vi "BuildConfigurationFilePaths.vi"(0 "name or relative path":string="Report Cummulative") -> (4 "Base Path":path=path "C:/Minda", 6 "User Configuration":path=path "C:/Minda/Configuration Files/UserConfiguration.usr", 8 "Product Configuration":path=path "C:/Minda/Configuration Files/ProductConfiguration.pdt", 10 "HWIO Configuration":path=path "C:/Minda/Configuration Files/HWIOConfiguration.txt", 14 "System File Path":path=path "C:/Minda/A-0090-System.bin" caption="System Verify")   [LabVIEW 2015]
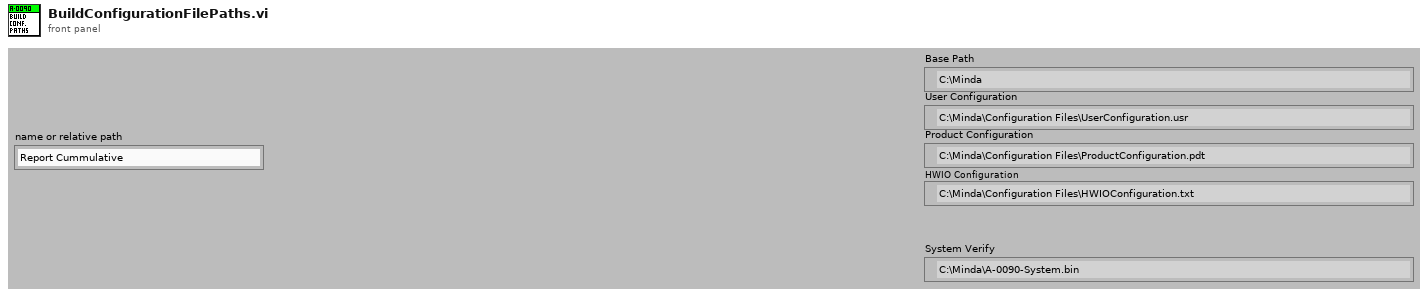
[diagram p1: front panel]
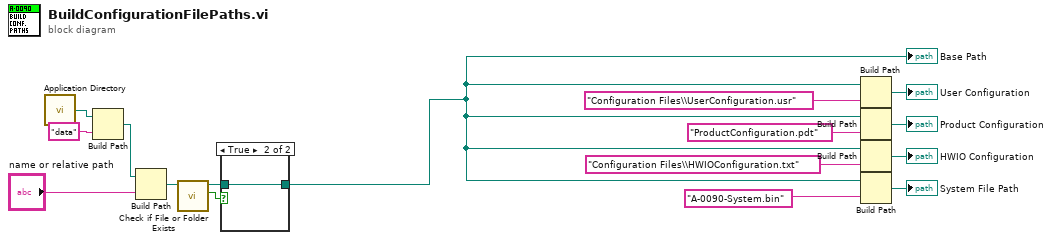
[diagram p0: block diagram]
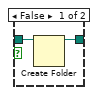
[diagram p2: hidden frame]
diagram:
  n1 = call <vilib>:"Application Directory.vi"() -> ("Application Directory"=w3:path)
  n2 = Build Path(base path=w3, name or relative path="data") -> (appended path=w2:path)
  n3 = Build Path(base path=w2, name or relative path="name or relative path") -> (appended path=w6:path)
  n4 = call <vilib>:"Check if File or Folder Exists.vi"("path"=w6) -> ("file or folder exists?"=w5:bool, "dup path"=w4:path)  [unwired: 8 in, 1 out]
  n5 = case shown="True" w5 {
    tunnel: w4 -> [w18 w19]
    tunnel: [w17 w19] -> w1
    frame False {
      n6 = Create Folder(path (use dialog)=w18) -> (created path=w17:path)  [unwired: 2 in, 2 out]
    }
    frame True {
    }
  }
  "Base Path" <- w1
  n7 = Build Path(base path=w1, name or relative path="Configuration Files\\UserConfiguration.usr" ("string")) -> (appended path=→"User Configuration":path)
  n8 = Build Path(base path=w1, name or relative path="ProductConfiguration.pdt" ("string")) -> (appended path=→"Product Configuration":path)
  n9 = Build Path(base path=w1, name or relative path="Configuration Files\\HWIOConfiguration.txt" ("string")) -> (appended path=→"HWIO Configuration":path)
  n10 = Build Path(base path=w1, name or relative path="A-0090-System.bin" ("string")) -> (appended path=→"System File Path":path)
